vi "SV Measure Delay and Polarity and Coherence.vi"(0 "reference signal":waveform(dbl)={"t0"=timestamp(0 s since 1904-01-01), "dt"=0.0, "Y"=[]}, 1 "ignore time stamp (T)":bool=TRUE, 5 "response signal":waveform(dbl)={"t0"=timestamp(0 s since 1904-01-01), "dt"=0.0, "Y"=[]}, 11 "error in":errorcluster) -> (3 "coherence":dbl format="%_4g", 4 "delay [s]":dbl format="%_4p", 6 "delay [samples]":dbl format="%_4f", 8 "polarity":dbl(ring) items=["Positive"=1.0, "Zero"=0.0, "Negative"=-1.0], 15 "error out":errorcluster)   [LabVIEW 2017, in "SoundVib_Calibration.lvlib"]
doc: "Use this VI to measure the propagation delay of a response signal. Use this VI when performing stimulus-response measurements to polarity normalize and time align the response signals prior to precision block processing. Use the equal polarity instance when the delayed signal exhibits equal polarity and simple time delay."
uses:
  <vilib>/addons/Sound and Vibration/svt_Calibration/SoundVib_Calibration.lvlib
  <vilib>/Analysis/_algsub.llb/Vector Norm Type.ctl
  <vilib>/Analysis/_algsub.llb/Real Vector Norm.vi
  <vilib>/addons/_NISVFA/_Shared subVIs/Common/svc_Get Array Subset (Index).vi
  <vilib>/addons/_NISVFA/_Shared subVIs/Common/svc_Coerce Index and Length.vi
  <vilib>/addons/_NISVFA/_Shared subVIs/Common/svc_Conditional Merge Error.vi
  <vilib>/Analysis/2dsp.llb/1D Cross Correlation (DBL).vi
  <vilib>/Analysis/NI_AALPro.lvlib
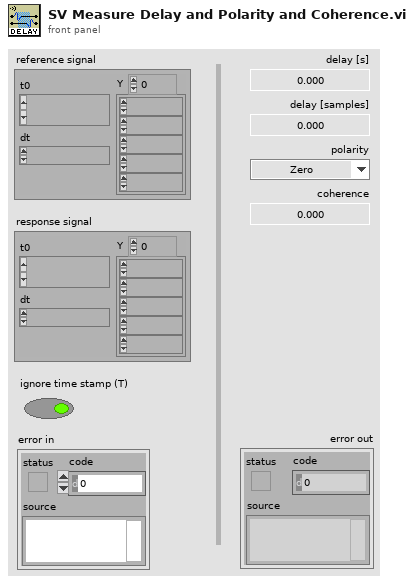
[diagram p1: front panel]
types:
  T1 = typedef "NI_AALPro.lvlib/Vector Norm Type.ctl" = u16
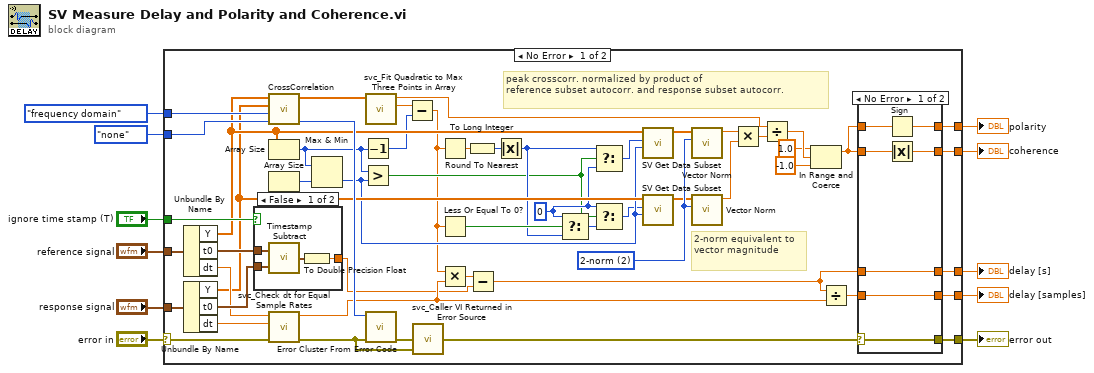
[diagram p0: block diagram]
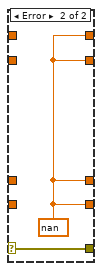
[diagram p2: hidden frame]
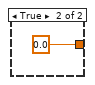
[diagram p3: hidden frame]
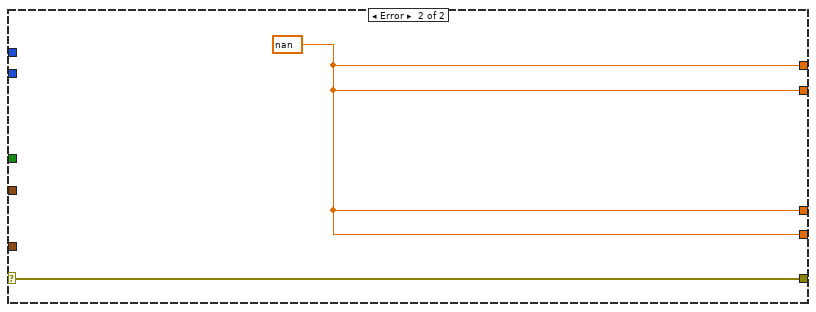
[diagram p4: hidden frame]
diagram:
  n1 = case shown="No Error" "error in" {
    selector: "error in" -> [w56 w79]
    tunnel: [w44 w79] -> w10
    tunnel: "response signal" -> [w50 _]
    tunnel: "reference signal" -> [w51 _]
    tunnel: enum32{"direct", "frequency domain"}."frequency domain" ("algorithm") -> [w61 _]
    tunnel: enum32{"none", "unbiased", "biased"}."none" ("normalization") -> [w60 _]
    tunnel: [w39 w78] -> w5
    tunnel: [w40 w78] -> w4
    tunnel: [w43 w78] -> w3
    tunnel: "ignore time stamp (T)" -> [w54 _]
    tunnel: [w41 w78] -> w1
    frame No Error {
      w22 = 0 ("start index")
      w33 = T1 2 items=["1-norm"=1, "2-norm"=2, "Inf-norm"=3, "-Inf-norm"=4, "User Defined"=5] ("norm type")
      # "2-norm equivalent to vector magnitude"
      # "peak crosscorr. normalized by product of \nreference subset autocorr. and response subset autocorr."
      n2 = Unbundle By Name(w51) -> ("Y"=w29:dbl[], "t0"=w49:timestamp, "dt"=w47:dbl)
      n3 = Unbundle By Name(w50) -> ("Y"=w28:dbl[], "t0"=w48:timestamp, "dt"=w46:dbl)
      n4 = case shown="False" w54 {
        tunnel: w49 -> [w75 _]
        tunnel: w48 -> [w74 _]
        tunnel: [w73 0.0] -> w32
        frame False {
          n5 = call <vilib>:"Timestamp Subtract.vi"("y"=w74, "x"=w75) -> ("x - y"=w76:timestamp)
          n6 = To Double Precision Float(number=w76) -> (double precision float=w73:dbl)
        }
        frame True {
        }
      }
      n7 = call-poly <vilib>:"CrossCorrelation.vi"("normalization"=w60, "algorithm"=w61, "Y"=w28, "X"=w29) -> ("error"=w63:i32, "Rxy"=w57:dbl[])  [unwired: 6 in]
      n8 = Array Size(array=w29) -> (size(s)=w17:i32)
      n9 = Array Size(array=w28) -> (size(s)=w37:i32)
      n10 = call <vilib>:"svc_Check dt for Equal Sample Rates.vi"("error in (no error)"=w56, "dt Y"=w46, "dt X"=w47) -> ("error out"=w55:errorcluster, "dt Y"=w52:dbl)  [unwired: 7 in]
      n11 = Max & Min(x=w17, y=w37) -> (min(x,y)=w25:i32)  [unwired: 1 out]
      n12 = Decrement(x=w17) -> (x-1=w15:i32)
      n13 = Greater?(x=w17, y=w25) -> (0:w18:bool)
      n14 = call <vilib>:"svc_Fit Quadratic to Max Three Points in Array.vi"("input array"=w57) -> ("fractional index"=w14:dbl, "y extreme"=w12:dbl)  [unwired: 9 in]
      n15 = call <vilib>:"Error Cluster From Error Code.vi"("error in (no error)"=w55, "error code (0)"=w63) -> ("error out"=w62:errorcluster)  [unwired: 7 in]
      n16 = Subtract(x=w14, y=w15) -> (x-y=w13:dbl)
      n17 = call <vilib>:"svc_Caller VI Returned in Error Source.vi"("warning input to caller"=w55, "error in (no error)"=w62) -> ("error out"=w45:errorcluster)  [unwired: 3 in]
      n18 = Round To Nearest(number=w13) -> (nearest integer value=w27:dbl)
      n19 = Less Or Equal To 0?(x=w13) -> (x <= 0?=w23:bool)
      n20 = Multiply(x=w13, y=w52) -> (x*y=w53:dbl)
      n21 = To Long Integer(number=w27) -> (32bit integer=w26:i32)
      n22 = Subtract(x=w53, y=w32) -> (x-y=w42:dbl)
      n23 = Absolute Value(x=w26) -> (abs(x)=w19:i32)
      n24 = Select(t=w22, s=w23, f=w19) -> (s? t:f=w21:i32)
      n25 = Select(t=w19, s=w18, f=w22) -> (s? t:f=w24:i32)
      n26 = Select(t=w22, s=w18, f=w21) -> (s? t:f=w20:i32)
      n27 = call-poly <vilib>:"SV Get Data Subset.vi"("length (-1 = all)"=w25, "start index (0)"=w24, "Y"=w29) -> ("Y subset"=w30:dbl[])  [unwired: 4 in, 4 out]
      n28 = call-poly <vilib>:"SV Get Data Subset.vi"("length (-1 = all)"=w25, "start index (0)"=w20, "Y"=w28) -> ("Y subset"=w31:dbl[])  [unwired: 4 in, 4 out]
      n29 = call-poly <vilib>:"Vector Norm.vi"("norm type"=w33, "Input Vector"=w30) -> ("norm"=w59:dbl)  [unwired: 8 in, 1 out]
      n30 = call-poly <vilib>:"Vector Norm.vi"("norm type"=w33, "Input Vector"=w31) -> ("norm"=w34:dbl)  [unwired: 8 in, 1 out]
      n31 = Multiply(x=w59, y=w34) -> (x*y=w36:dbl)
      n32 = Divide(x=w12, y=w36) -> (x/y=w58:dbl)
      n33 = In Range and Coerce(upper limit=1.0, x=w58, lower limit=-1.0 ("upper limit")) -> (coerced(x)=w38:dbl)  [unwired: 1 out]
      n34 = Divide(x=w42, y=w52) -> (x/y=w43:dbl)
      n35 = case shown="No Error" w45 {
        selector: w45 -> [w70 w72]
        tunnel: [w70 w72] -> w44
        tunnel: [w69 w71] -> _
        tunnel: w43 -> [w69 _]
        tunnel: [w68 w71] -> w41
        tunnel: w42 -> [w68 _]
        tunnel: [w64 w71] -> w40
        tunnel: [w66 w71] -> w39
        tunnel: w38 -> [w67 _]
        tunnel: w38 -> [w65 _]
        frame No Error {
          n36 = Sign(1:w67) -> (0:w66:dbl)
          n37 = Absolute Value(x=w65) -> (abs(x)=w64:dbl)
        }
        frame Error {
          w71 = nan ("lower limit")
        }
      }
    }
    frame Error {
      w78 = nan
    }
  }
  "error out" <- w10
  "polarity" <- w5
  "coherence" <- w4
  "delay [s]" <- w1
  "delay [samples]" <- w3
